vi "LEDSOnGlobal.vi"() -> ()   [LabVIEW 2019]
panel:
  in  "LEDs On":bool
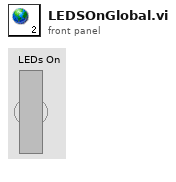
[diagram p1: front panel]
diagram:
